vi "Simple PID.vi"(1 "Saturation":dbl[](array[numeric])=[-1.0, 1.0], 2 "Position":dbl, 3 "Reference":dbl, 4 "PID Gains":cluster{"Kp":dbl, "Kd":dbl, "Ki":dbl}) -> (0 "Output":dbl)   [LabVIEW 2018]
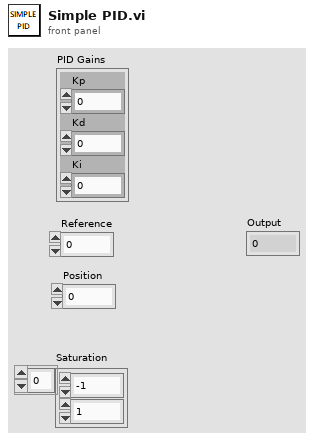
[diagram p1: front panel]
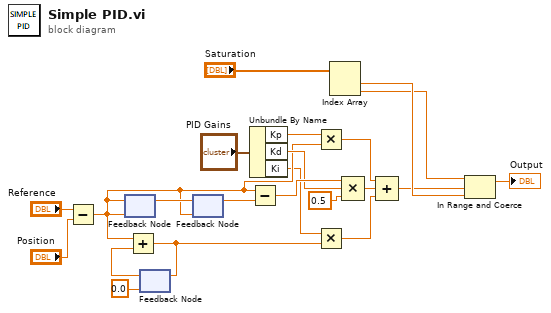
[diagram p0: block diagram]
diagram:
  n1 = Subtract(x="Reference", y="Position") -> (x-y=w11:dbl)
  n2 = feedback #1(w11) -> (w17:dbl)
  n3 = feedback-in #1(w11) -> ()
  n4 = feedback #2(0.0 ("value")) -> (w10:dbl)
  n5 = Add(x=w11, y=w10) -> (x+y=w7:dbl)
  n6 = feedback-in #2(w7) -> ()
  n7 = feedback #3(w11) -> (w16:dbl)
  n8 = feedback-in #3(w17) -> ()
  n9 = Unbundle By Name("PID Gains") -> ("Kp"=w19:dbl, "Kd"=w14:dbl, "Ki"=w8:dbl)
  n10 = Subtract(x=w11, y=w16) -> (x-y=w15:dbl)
  n11 = Multiply(x=w19, y=w11) -> (x*y=w18:dbl)
  n12 = Multiply(x=w8, y=w7) -> (x*y=w6:dbl)
  n13 = Index Array(array="Saturation") -> (element #1=w4:dbl, element #2=w3:dbl)  [unwired: 2 in]
  n14 = Compound Arithmetic op=MULTIPLY(w15, w14, 0.5 ("value")) -> (w12:dbl)
  n15 = Compound Arithmetic op=ADD(w18, w12, w6) -> (w2:dbl)
  n16 = In Range and Coerce(upper limit=w3, x=w2, lower limit=w4) -> (coerced(x)=→"Output":dbl)  [unwired: 1 out]
